vi "BD Timestamp to Labview TimeStamp.vi"(2 "error in":errorcluster, 3 "BD Time Stamp":string) -> (0 "error out":errorcluster, 1 "time stamp":timestamp)   [LabVIEW 2020, in "PostgreSQL Driver.lvlib"]
uses:
  PostgreSQL Driver.lvlib
  <vilib>/Utility/miscctls.llb/LVDateTimeRec.ctl
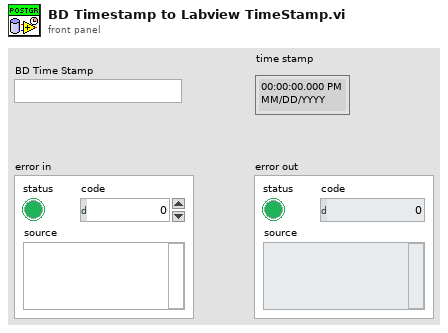
[diagram p1: front panel]
types:
  T1 = typedef "LVDateTimeRec.ctl" = cluster{"fractional second":dbl, "second":i32, "minute":i32, "hour":i32, "day of month":i32, "month":i32, "year":i32, "day of week":i32, "day of year":i32, "DST":i32}
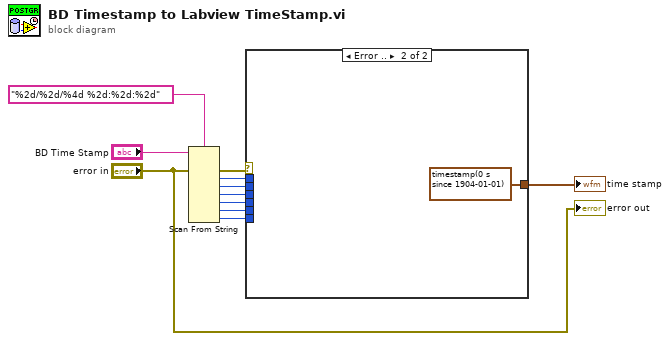
[diagram p0: block diagram]
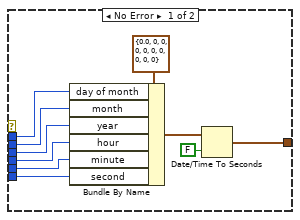
[diagram p2: hidden frame]
diagram:
  n1 = Scan From String(format string="%2d/%2d/%4d %2d:%2d:%2d", input string="BD Time Stamp", error in="error in") -> (error out=w2:errorcluster, output 1=w9:i32, output 2=w8:i32, output 3=w7:i32, output 4=w3:i32, output 5=w6:i32, output 6=w5:i32)  [unwired: 7 in, 2 out]
  n2 = case shown="Error .." w2 {
    tunnel: w9 -> [w19 _]
    tunnel: w8 -> [w18 _]
    tunnel: w7 -> [w17 _]
    tunnel: w6 -> [w16 _]
    tunnel: w5 -> [w15 _]
    tunnel: [w14 timestamp(0 s since 1904-01-01) ("time stamp")] -> w4
    tunnel: w3 -> [w12 _]
    frame No Error {
      n3 = Bundle By Name(cluster=T1 {"fractional second"=0.0, "second"=0, "minute"=0, "hour"=0, "day of month"=0, "month"=0, "year"=0, "day of week"=0, "day of year"=0, "DST"=0} ("date time rec"), "day of month"=w19, "month"=w18, "year"=w17, "hour"=w12, "minute"=w16, "second"=w15) -> (w21:T1)
      n4 = Date/Time To Seconds(1:FALSE ("is UTC (F)"), 2:w21) -> (0:w14:timestamp)
    }
    frame Error {
    }
  }
  "time stamp" <- w4
  "error out" <- "error in"
